vi "Robot Drive Direct.vi"(8 "error in":errorcluster, 9 "Left Wheel Velocity (mm/s)":i16, 10 "Right Wheel Velocity (mm/s)":i16, 11 "UART port in":refnum<visa-resource-name>) -> (0 "error out":errorcluster, 3 "UART port out":refnum<visa-resource-name>)   [LabVIEW 2014]
doc: "Directly actuate left and right wheels.\n\nThis VI writes to, but does not read from, the serial port."
uses:
  Kobuki/Kobuki_cmdID.ctl
panel:
  out "appended array":cluster{"Max Speed (mm/s)":i16, "radius":i16}[](array[cluster])
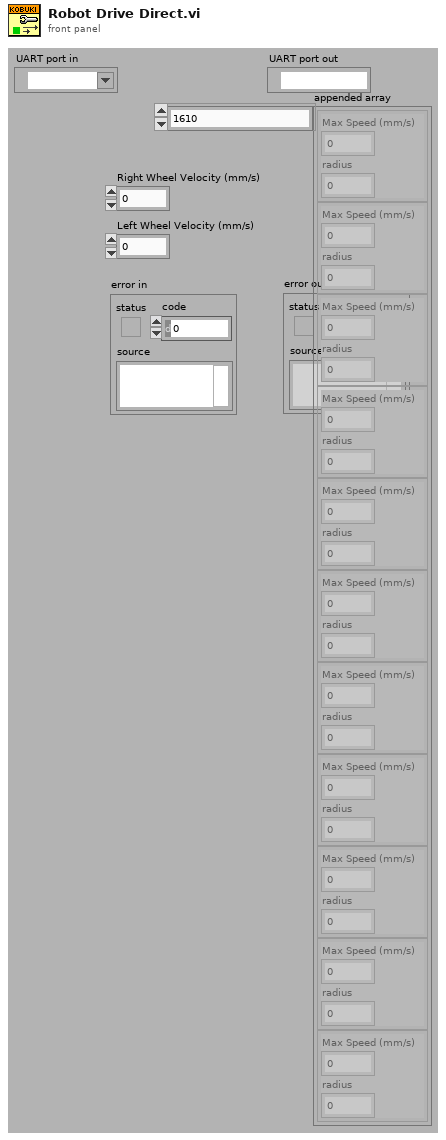
[diagram p1: front panel]
types:
  T1 = typedef "Kobuki_cmdID.ctl" = u8
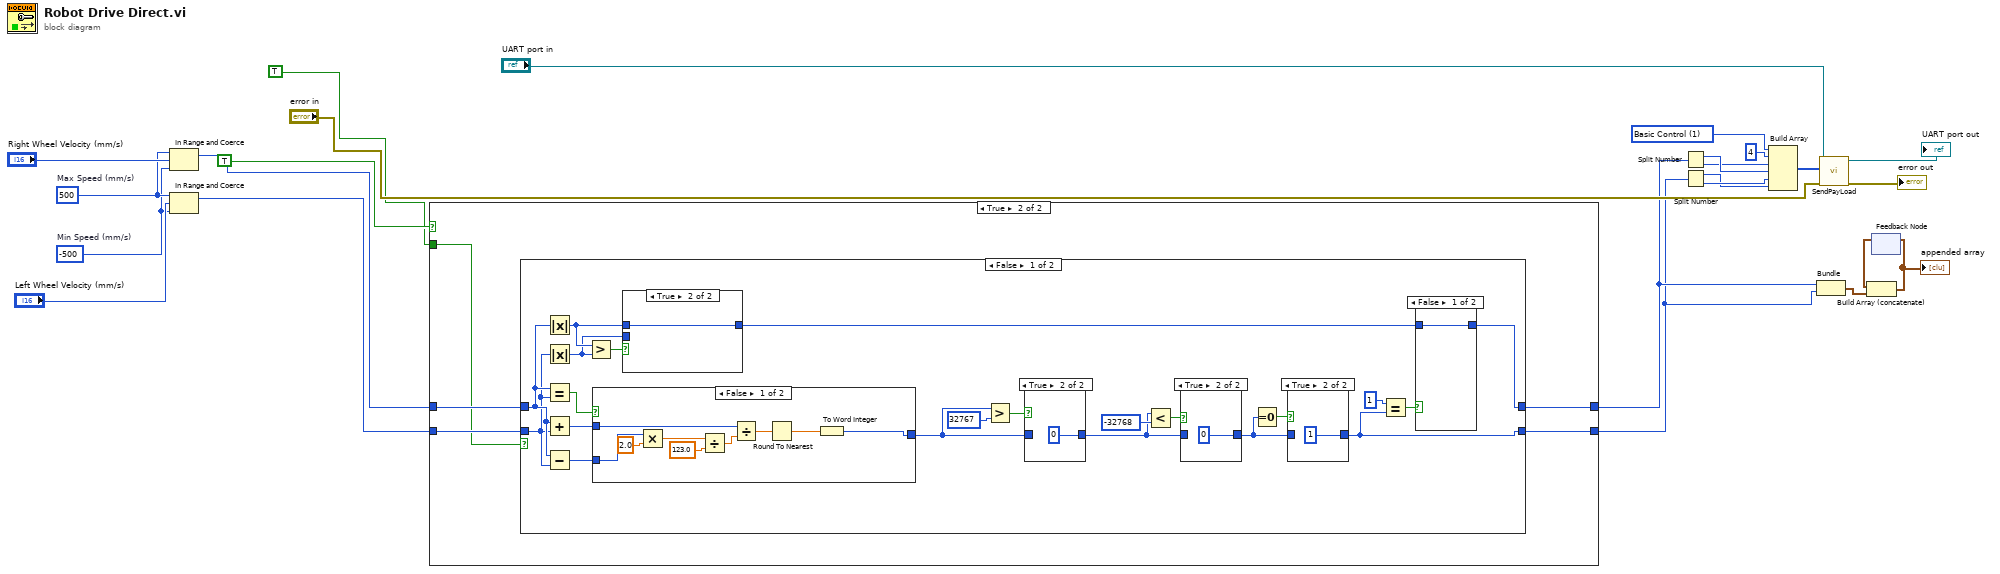
[diagram p0: block diagram]
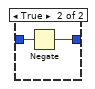
[diagram p3: hidden frame]
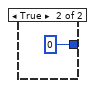
[diagram p7: hidden frame]
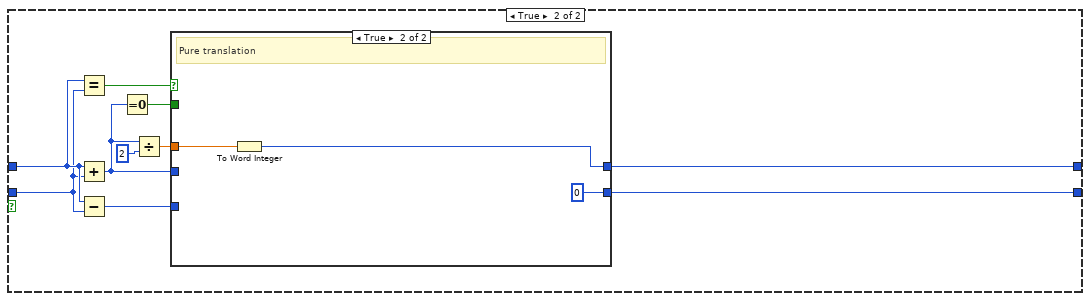
[diagram p9: hidden frame]
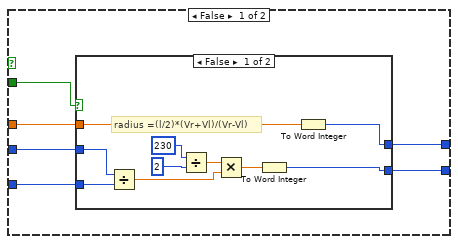
[diagram p10: hidden frame]
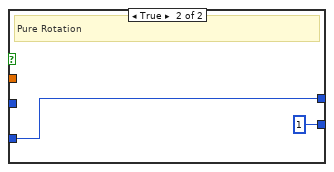
[diagram p11: hidden frame]
diagram:
  w8 = T1 1 items=["Basic Control"=1, "Sound"=3, "Sound Sequence"=4, "Request Extra"=9, "General Purpose Output"=12, "Set Controller Gain"=13, "Get Controller Gain"=14] ("Command Packets ID")
  w21 = i16 -500  # Min Speed (mm/s)
  w22 = i16 500  # Max Speed (mm/s)
  n1 = In Range and Coerce(upper limit=w22, x="Right Wheel Velocity (mm/s)", lower limit=w21) -> (coerced(x)=w18:i16)  [unwired: 1 out]
  n2 = In Range and Coerce(upper limit=w22, x="Left Wheel Velocity (mm/s)", lower limit=w21) -> (coerced(x)=w17:i16)  [unwired: 1 out]
  n3 = case shown="True" TRUE ("KobukiDriveDirect?") {
    tunnel: [w25 w31] -> w4
    tunnel: [w26 w30] -> w5
    tunnel: w18 -> [w26 w29]
    tunnel: w17 -> [w25 w28]
    tunnel: TRUE ("Boolean") -> [_ w27]
    frame False {
    }
    frame True {
      n4 = case shown="False" w27 {
        tunnel: [w34 w82] -> w31
        tunnel: [w32 w81] -> w30
        tunnel: w29 -> [w46 w77]
        tunnel: w28 -> [w45 w76]
        frame False {
          n5 = Absolute Value(x=w46) -> (abs(x)=w52:i16)
          n6 = Absolute Value(x=w45) -> (abs(x)=w51:i16)
          n7 = Equal?(x=w46, y=w45) -> (x = y?=w49:bool)
          n8 = Add(x=w46, y=w45) -> (x+y=w48:i16)
          n9 = Subtract(x=w46, y=w45) -> (x-y=w47:i16)
          n10 = Greater?(x=w52, y=w51) -> (0:w50:bool)
          n11 = case shown="False" w49 {
            tunnel: [w62 i16 0] -> w42
            tunnel: w48 -> [w70 _]
            tunnel: w47 -> [w68 _]
            frame False {
              n12 = Multiply(x=w68, y=2.0) -> (x*y=w67:dbl)
              n13 = Divide(x=w67, y=123.0) -> (x/y=w65:dbl)
              n14 = Divide(x=w70, y=w65) -> (x/y=w64:dbl)
              n15 = Round To Nearest(number=w64) -> (nearest integer value=w63:dbl)
              n16 = To Word Integer(number=w63) -> (16bit integer=w62:i16)
            }
            frame True {
            }
          }
          n17 = case shown="True" w50 {
            tunnel: [w72 w73] -> w33
            tunnel: w52 -> [_ w73]
            tunnel: w51 -> [w72 _]
            frame False {
            }
            frame True {
            }
          }
          n18 = Greater?(x=w42, y=i16 32767) -> (0:w44:bool)
          n19 = case shown="True" w44 {
            tunnel: w42 -> [w60 _]
            tunnel: [w60 i16 0] -> w37
            frame False {
            }
            frame True {
            }
          }
          n20 = Less?(x=w37, y=i16 -32768) -> (x < y?=w40:bool)
          n21 = case shown="True" w40 {
            tunnel: w37 -> [w58 _]
            tunnel: [w58 i16 0] -> w39
            frame False {
            }
            frame True {
            }
          }
          n22 = Equal To 0?(x=w39) -> (x = 0?=w38:bool)
          n23 = case shown="True" w38 {
            tunnel: w39 -> [w56 _]
            tunnel: [w56 i16 1] -> w34
            frame False {
            }
            frame True {
            }
          }
          n24 = Equal?(x=i16 1, y=w34) -> (x = y?=w35:bool)
          n25 = case shown="False" w35 {
            tunnel: w33 -> [w53 w55]
            tunnel: [w53 w54] -> w32
            frame False {
            }
            frame True {
              n26 = Negate(x=w55) -> (-x=w54:i16)
            }
          }
        }
        frame True {
          n27 = Equal?(x=w77, y=w76) -> (x = y?=w83:bool)
          n28 = Add(x=w77, y=w76) -> (x+y=w74:i16)
          n29 = Subtract(x=w77, y=w76) -> (x-y=w75:i16)
          n30 = Equal To 0?(x=w74) -> (x = 0?=w80:bool)
          n31 = Divide(x=w74, y=i16 2) -> (x/y=w78:dbl)
          n32 = case shown="True" w83 {
            tunnel: [w88 i16 0 ("radius")] -> w82
            tunnel: [w87 w102] -> w81
            tunnel: w80 -> [w89 _]
            tunnel: w78 -> [w86 w103]
            tunnel: w75 -> [w84 _]
            tunnel: w74 -> [w85 _]
            frame False {
              n33 = case shown="False" w89 {
                tunnel: [w94 i16 1 ("radius")] -> w88
                tunnel: [w92 w100] -> w87
                tunnel: w86 -> [w93 _]
                tunnel: w85 -> [w91 _]
                tunnel: w84 -> [w90 w100]
                frame False {
                  # "radius =(l/2)*(Vr+Vl)/(Vr-Vl)"
                  n34 = Divide(x=w91, y=w90) -> (x/y=w96:dbl)
                  n35 = Divide(x=i16 230, y=i16 2) -> (x/y=w97:dbl)
                  n36 = Multiply(x=w97, y=w96) -> (x*y=w95:dbl)
                  n37 = To Word Integer(number=w95) -> (16bit integer=w94:i16)
                  n38 = To Word Integer(number=w93) -> (16bit integer=w92:i16)
                }
                frame True {
                  # "Pure Rotation"
                }
              }
            }
            frame True {
              # "Pure translation"
              n39 = To Word Integer(number=w103) -> (16bit integer=w102:i16)
            }
          }
        }
      }
    }
  }
  n40 = Split Number(x=w5) -> (hi(x)=w13:u8, lo(x)=w9:u8)
  n41 = Split Number(x=w4) -> (hi(x)=w11:u8, lo(x)=w12:u8)
  n42 = Build Array(w8, u8 4, w9, w13, w12, w11) -> (w10:T1[])
  n43 = Bundle("Max Speed (mm/s)"=w5, "radius"=w4) -> (w3:cluster{"Max Speed (mm/s)":i16, "radius":i16})  [unwired: 1 in]
  n44 = call "SendPayLoad.vi"("error in (no error)"="error in", "PayLoad"=w10, "VISA Refnum in"="UART port in") -> ("error out"=→"error out":errorcluster, "VISA Refnum out"=→"UART port out":refnum<visa-resource-name>)  [unwired: 7 in]
  n45 = feedback #1() -> (w1:cluster{"Max Speed (mm/s)":i16, "radius":i16}[])  [unwired: 1 in]
  n46 = Build Array (concatenate)(w1, w3) -> (w2:cluster{"Max Speed (mm/s)":i16, "radius":i16}[])
  "appended array" <- w2
  n47 = feedback-in #1(w2) -> ()
